vi "Mining and Dumping_r2.vi"() -> ()   [LabVIEW 2015]
uses:
  <vilib>/myRIO/Instrument Drivers/Onboard IO/PWM/typedefs/PWM Reference.ctl
  <vilib>/myRIO/Common/Instrument Driver Framework/Utilities/typedefs/myRIO Generic Hardware Reference.ctl
  <vilib>/myRIO/Common/Instrument Driver Framework/Utilities/typedefs/Hardware Version Enum.ctl
  <vilib>/myRIO/Common/Instrument Driver Framework/Utilities/typedefs/myRIO v1.0 Reference.ctl
  <vilib>/myRIO/Common/Instrument Driver Framework/Utilities/typedefs/Generic FPGA Reference.ctl
  <vilib>/myRIO/Common/Instrument Driver Framework/myRIO v1.0/PWM/typedefs/PWM Channels Enum.ctl
  <vilib>/myRIO/Instrument Drivers/Onboard IO/PWM/typedefs/PWM Configuration.ctl
  <vilib>/userdefined/High Color/nirio_resource_hc.ctl
  <vilib>/myRIO/Instrument Drivers/Onboard IO/AI/typedefs/AI Reference.ctl
  <vilib>/myRIO/Common/Instrument Driver Framework/myRIO v1.0/AI/typedefs/AI Channels List.ctl
  <vilib>/myRIO/Common/Instrument Driver Framework/myRIO v1.0/AI/typedefs/AI Channels Enum.ctl
  <vilib>/myRIO/Common/Instrument Driver Framework/Utilities/typedefs/Analog Scaling Constants List.ctl
  <vilib>/myRIO/Common/Instrument Driver Framework/Utilities/typedefs/Analog Scaling Constants.ctl
  <vilib>/myRIO/Common/Instrument Driver Framework/Utilities/vis/Is FPGA Ref Available.vi
  <vilib>/myRIO/Common/Instrument Driver Framework/myRIO v1.0/PWM/vis/myRIO v1.1 Open PWM.vi
  <vilib>/myRIO/Instrument Drivers/Onboard IO/PWM/vis/Set Duty Cycle and Frequency.vi
  <vilib>/myRIO/Common/Instrument Driver Framework/myRIO v1.0/AI/vis/myRIO v1.1 Open AI.vi
  <vilib>/myRIO/Instrument Drivers/Onboard IO/AI/vis/Read.vi
  <vilib>/myRIO/Common/Instrument Driver Framework/Utilities/vis/Validate Channels.vi
  <vilib>/myRIO/Common/Instrument Driver Framework/myRIO v1.0/PWM/vis/myRIO v1.0 Reserve PWM.vi
  <vilib>/myRIO/Common/Instrument Driver Framework/myRIO v1.0/AI/vis/myRIO v1.0 Reserve AI.vi
  <vilib>/myRIO/Common/Instrument Driver Framework/myRIO v1.0/PWM/vis/myRIO v1.0 Build MUX Configuration PWM.vi
  <vilib>/myRIO/Common/Instrument Driver Framework/myRIO v1.0/Resource Manager/vis/myRIO v1.0 Reserve Channel List.vi
  <vilib>/myRIO/Common/Instrument Driver Framework/myRIO v1.0/AI/vis/myRIO v1.0 Build MUX Configuration AI.vi
  <vilib>/myRIO/Common/Instrument Driver Framework/myRIO v1.0/Resource Manager/vis/myRIO v1.0 Create Configuration List.vi
  <vilib>/myRIO/Common/Instrument Driver Framework/myRIO v1.0/Resource Manager/vis/myRIO v1.0 Reserve Channel.vi
  <vilib>/myRIO/Common/Instrument Driver Framework/myRIO v1.0/Resource Manager/vis/myRIO v1.0 Unreserve Channel.vi
  <vilib>/myRIO/Common/Instrument Driver Framework/myRIO v1.0/Resource Manager/vis/myRIO v1.0 Build Mutex Name.vi
  <vilib>/Utility/VariantDataType/GetNumericInfo.vi
  <vilib>/Utility/error.llb/Error Cluster From Error Code.vi
  <vilib>/myRIO/Common/Instrument Driver Framework/myRIO v1.0/myRIO v1.1 Open.vi
  <vilib>/myRIO/Common/Instrument Driver Framework/Utilities/vis/IO Manager.vi
  <vilib>/myRIO/Common/Instrument Driver Framework/Utilities/vis/Configuration Manager.vi
  <vilib>/myRIO/Common/Instrument Driver Framework/myRIO v1.0/Resource Manager/vis/myRIO v1.0 Configure IO.vi
  <vilib>/myRIO/Common/Instrument Driver Framework/myRIO v1.0/myRIO v1.0 Close.vi
  <vilib>/myRIO/Common/Instrument Driver Framework/myRIO v1.0/PWM/vis/myRIO v1.0 Write PWM.vi
  <vilib>/myRIO/Common/Instrument Driver Framework/myRIO v1.0/AI/vis/myRIO v1.0 Get Scaling Constants AI.vi
  <vilib>/myRIO/Common/Instrument Driver Framework/myRIO v1.0/AI/vis/myRIO v1.0 Read AI.vi
  <vilib>/myRIO/Express VI/Onboard IO/PWM/PWM Express VI.xnode
  <vilib>/myRIO/Instrument Drivers/Onboard IO/PWM/vis/myRIO PWM Open.xnode
  <vilib>/myRIO/Express VI/Onboard IO/AI/AI Express VI.xnode
  <vilib>/myRIO/Instrument Drivers/Onboard IO/AI/vis/myRIO AI Open.xnode
  <vilib>/myRIO/Instrument Drivers/Onboard IO/PWM/PWM.lvlib
  <vilib>/myRIO/Instrument Drivers/Onboard IO/AI/AI.lvlib
panel:
  in  "Stop":bool
  out "Servo Positioin 2":dbl
  out "Servo Position 1":dbl
  out "Servo Stop":i64
  out "Stop Mining":bool
  in  "Numeric":i32
  out "Full":bool
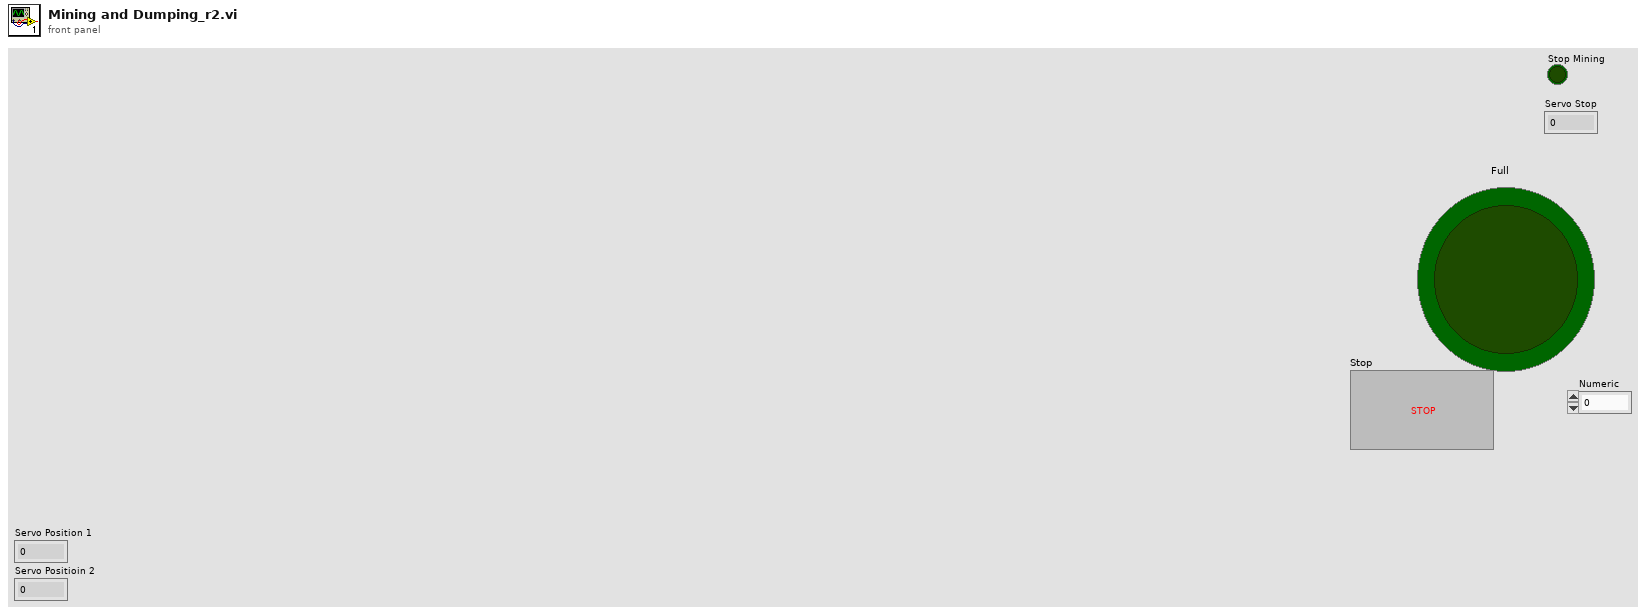
[diagram p1: front panel]
types:
  T1 = typedef "PWM.lvlib/PWM Reference.ctl" = cluster{"myRIO Reference":T2, "PWM Channels Enum":T6, "PWM Configuration":T7}
  T2 = typedef "myRIO Generic Hardware Reference.ctl" = cluster{"myRIO Model":T3, "myRIO Hardware Reference":T4}
  T3 = typedef "Hardware Version Enum.ctl" = enum16{"Unknown", "myRIO-1900", "myRIO-1950", "roboRIO"}
  T4 = typedef "myRIO v1.0 Reference.ctl" = cluster{"Generic FPGA Reference":T5, "Allow multiple opens":bool}
  T5 = typedef "Generic FPGA Reference.ctl" = refnum<k20>
  T6 = typedef "PWM Channels Enum.ctl" = enum16{"Not Connected", "C/PWM0", "C/PWM1", "A/PWM0", "A/PWM1", "A/PWM2", "B/PWM0", "B/PWM1", "B/PWM2", "PWM/PWM0", "PWM/PWM1", "PWM/PWM2", "PWM/PWM3", "PWM/PWM4", "PWM/PWM5", "PWM/PWM6", "PWM/PWM7", "PWM/PWM8", "PWM/PWM9"}
  T7 = typedef "PWM.lvlib/PWM Configuration.ctl" = cluster{"Frequency":dbl, "Duty Cycle":dbl}
  T8 = typedef "nirio_resource_hc.ctl" = tag
  T9 = typedef "AI.lvlib/AI Reference.ctl" = cluster{"myRIO Reference":T2, "AI Channels List":T10, "AI Scaling Constants List":T12}
  T10 = typedef "AI Channels List.ctl" = T11[]
  T11 = typedef "AI Channels Enum.ctl" = enum16{"Not Connected", "AudioIn/Left", "AudioIn/Right", "C/AI0", "C/AI1", "A/AI0", "A/AI1", "A/AI2", "A/AI3", "B/AI0", "B/AI1", "B/AI2", "B/AI3", "AI/AI0", "AI/AI1", "AI/AI2", "AI/AI3"}
  T12 = typedef "Analog Scaling Constants List.ctl" = T13[]
  T13 = typedef "Analog Scaling Constants.ctl" = cluster{"LSB Weight (Volts)":dbl, "Offset (Volts)":dbl, "Signed?":bool}
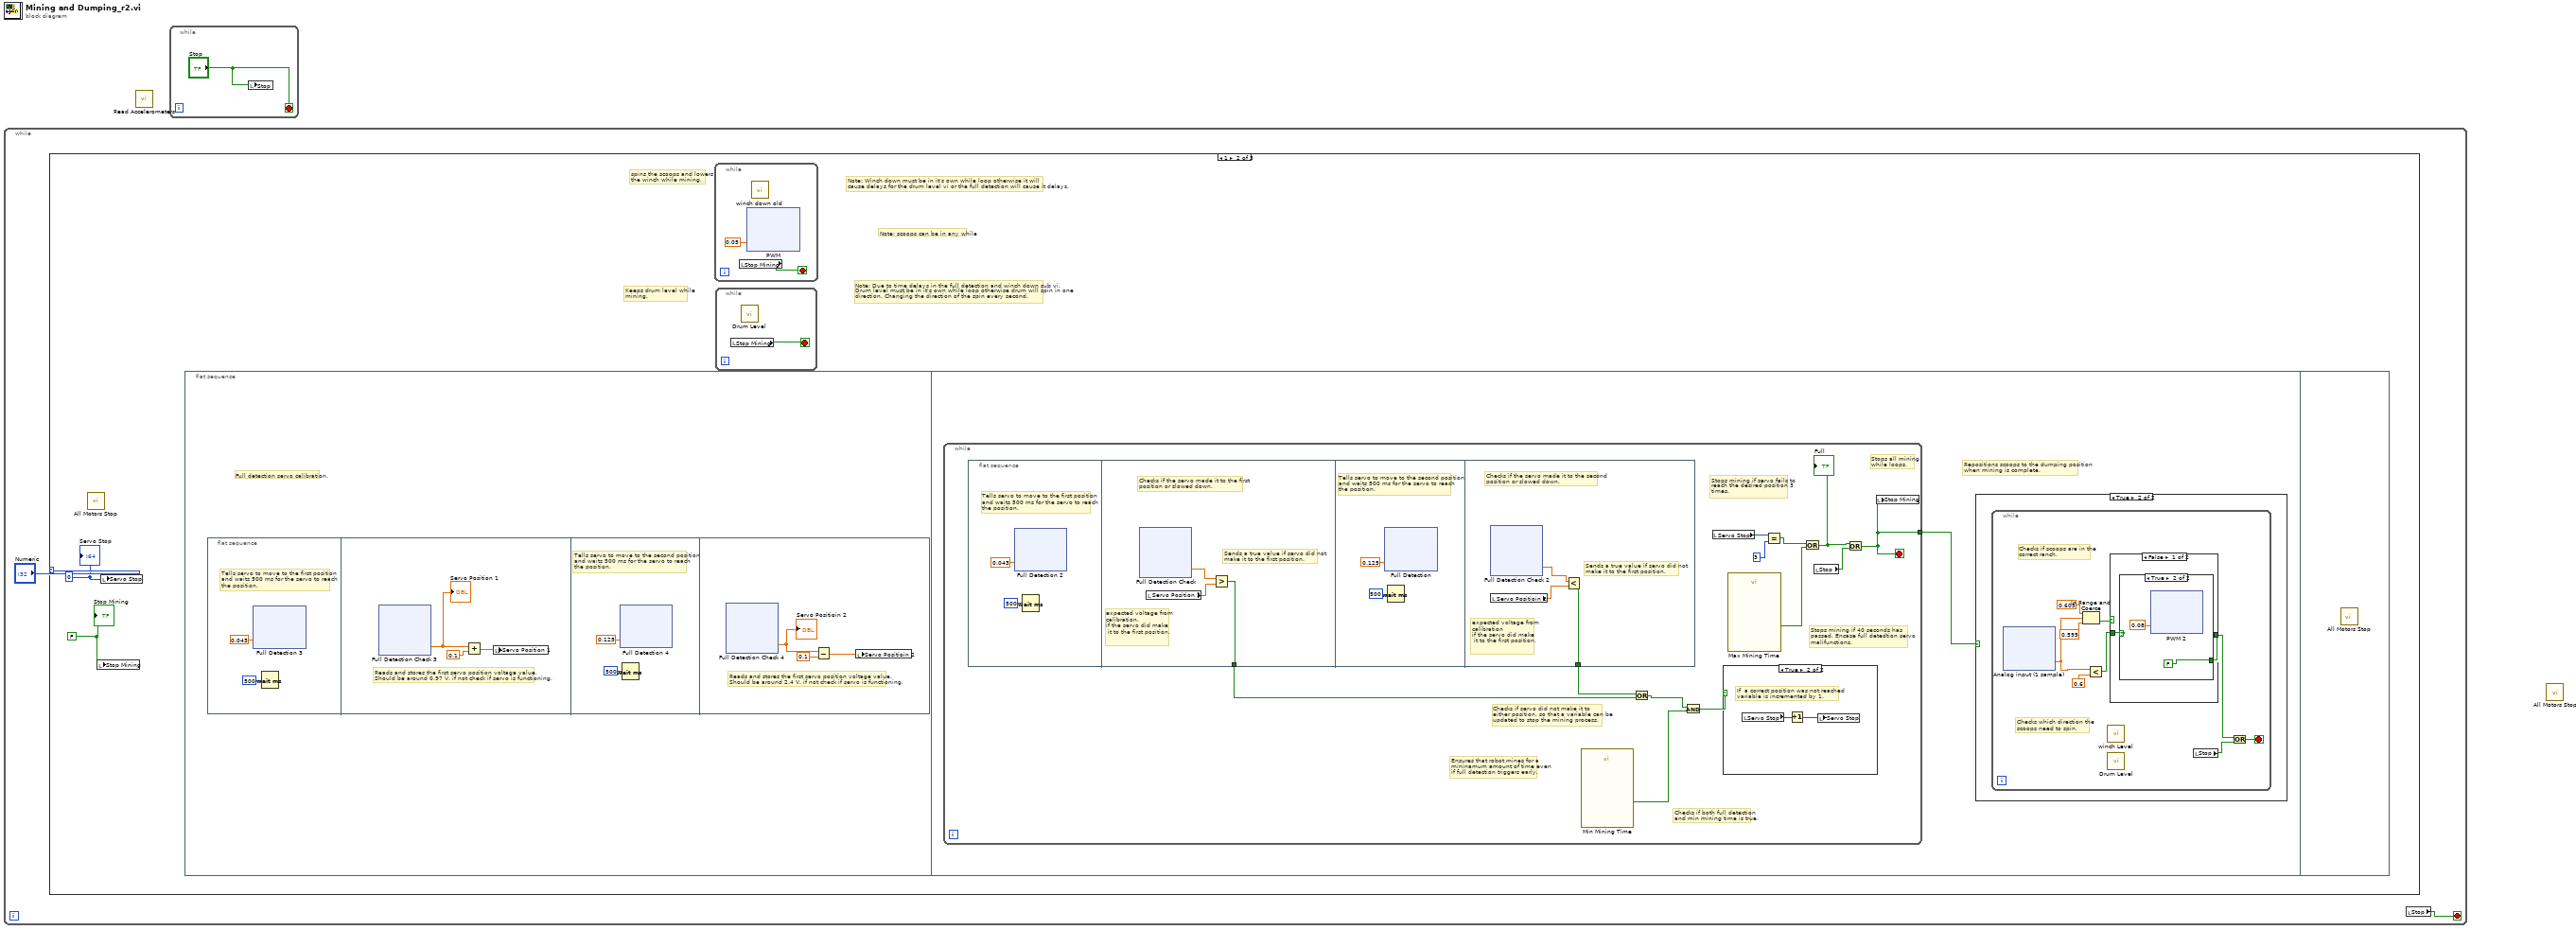
[diagram p0: block diagram]
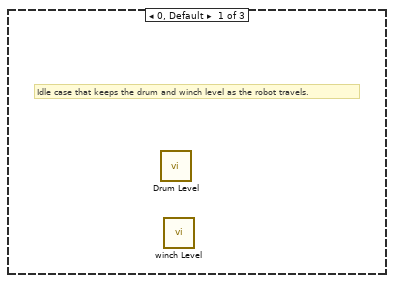
[diagram p2: hidden frame]
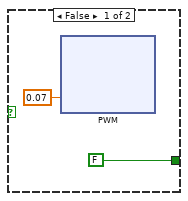
[diagram p4: hidden frame]
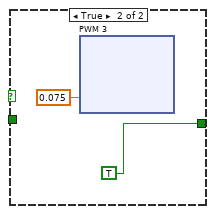
[diagram p5: hidden frame]
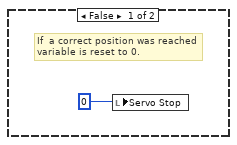
[diagram p6: hidden frame]
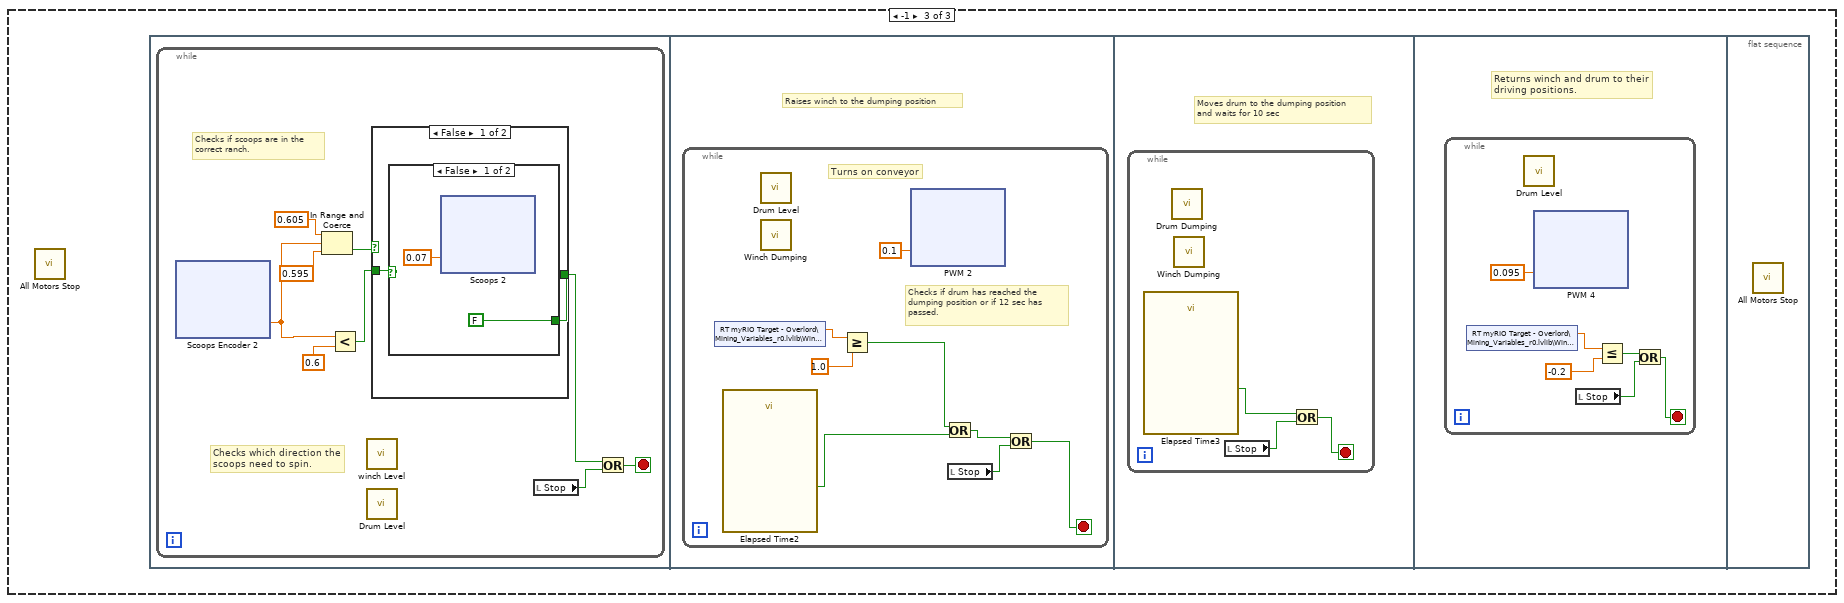
[diagram p7: hidden frame]
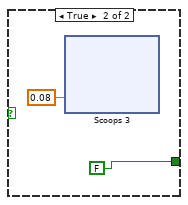
[diagram p8: hidden frame]
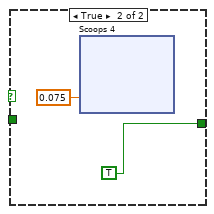
[diagram p9: hidden frame]
diagram:
  n1 = while {
    stop <- w1 stop-if-true
    n2 = case shown="1" "Numeric" {
      frame 0, Default {
        # "Idle case that keeps the drum and winch level as the robot travels."
        n3 = call "Drum Level.vi"() -> ()  [unwired: 12 in]
        n4 = call "winch Level.vi"() -> ()  [unwired: 12 in]
      }
      frame 1 {
        w4 = FALSE ("Stop")
        w3 = i64 0 ("Servo Stop")
        # "Note: scoops can be in any while"
        # "Note: Winch down must be in it's own while loop otherwise it will \ncause delays for the drum level vi or the full detection will cause it delays."
        # "Note: Due to time delays in the full detection and winch down sub vi.\nDrum level must be in it's own while loop otherwise drum will spin in one\ndirection. Changing the direction of the spin every second."
        # "spins the scoops and lowers\nthe winch while mining."
        # "Keeps drum level while \nmining."
        n5 = call "All Motors Stop.vi"() -> ()  [unwired: 12 in]
        n6 = local write "Stop Mining"(w4) -> ()
        n7 = local write "Servo Stop"(w3) -> ()
        n8 = flat-sequence {
          frame #0 {
            # "Full detection servo calibration."
            n9 = flat-sequence {
              frame #0 {
                # "Tells servo to move to the first position\nand waits 500 ms for the servo to reach \nthe position."
                n10 = xnode "Full Detection 3"("Duty Cycle"=0.043) -> ()  [unwired: 1 in, 1 out]
                n11 = Wait (ms)(milliseconds to wait=u32 500) -> ()  [unwired: 1 out]
              }
              frame #1 {
                # "Reads and stores the first servo position voltage value. \nShould be around 0.97 V. if not check if servo is functioning."
                n12 = xnode "Full Detection Check 3"() -> ("A/AI0 (Pin 3)"=w80:dbl)  [unwired: 1 in, 1 out]
                "Servo Position 1" <- w80
                n13 = Add(x=w80, y=0.1) -> (x+y=w81:dbl)
                n14 = local write "Servo Position 1"(w81) -> ()
              }
              frame #2 {
                # "Tells servo to move to the second position\nand waits 500 ms for the servo to reach \nthe position."
                n15 = xnode "Full Detection 4"("Duty Cycle"=0.125) -> ()  [unwired: 1 in, 1 out]
                n16 = Wait (ms)(milliseconds to wait=u32 500) -> ()  [unwired: 1 out]
              }
              frame #3 {
                # "Reads and stores the first servo position voltage value. \nShould be around 2.4 V. if not check if servo is functioning."
                n17 = xnode "Full Detection Check 4"() -> ("A/AI0 (Pin 3)"=w157:dbl)  [unwired: 1 in, 1 out]
                "Servo Positioin 2" <- w157
                n18 = Subtract(x=w157, y=0.1) -> (x-y=w158:dbl)
                n19 = local write "Servo Positioin 2"(w158) -> ()
              }
            }
          }
          frame #1 {
            # "Repositions scoops to the dumping position\nwhen mining is complete."
            n20 = while {
              tunnel: [w357] -> w196
              stop <- w357 stop-if-true
              # "Stops all mining \nwhile loops."
              # "Stops mining if 40 seconds has \npassed. Encase full detedtion servo \nmalifunctions."
              # "Stops mining if servo fails to \nreach the desired position 3\ntimes."
              # "Checks if both full detection \nand min mining time is true."
              # "Ensures that robot mines for a \nmininamum amount of time even\nif full detection triggers early."
              # "Checks if servo did not make it to\neither position. so that a variable can be \nupdated to stop the mining process."
              n21 = flat-sequence {
                tunnel: [w410] -> w366
                tunnel: [w486] -> w367
                frame #0 {
                  # "Tells servo to move to the first position\nand waits 500 ms for the servo to reach \nthe position."
                  n22 = xnode "Full Detection 2"("Duty Cycle"=0.043) -> ()  [unwired: 1 in, 1 out]
                  n23 = Wait (ms)(milliseconds to wait=u32 500) -> ()  [unwired: 1 out]
                }
                frame #1 {
                  # "Sends a true value if servo did not \nmake it to the first position."
                  # "expected voltage from \ncalibration.\nif the servo did make\n it to the first position."
                  # "Checks if the servo made it to the first \nposition or slowed down."
                  n24 = xnode "Full Detection Check"() -> ("A/AI0 (Pin 3)"=w409:dbl)  [unwired: 1 in, 1 out]
                  n25 = local read "Servo Position 1"() -> (w408:dbl)
                  n26 = Greater?(x=w409, y=w408) -> (0:w410:bool)
                }
                frame #2 {
                  # "Tells servo to move to the second position\nand waits 500 ms for the servo to reach \nthe position."
                  n27 = xnode "Full Detection"("Duty Cycle"=0.125) -> ()  [unwired: 1 in, 1 out]
                  n28 = Wait (ms)(milliseconds to wait=u32 500) -> ()  [unwired: 1 out]
                }
                frame #3 {
                  # "Sends a true value if servo did not \nmake it to the first position."
                  # "expected voltage from \ncalibration\nif the servo did make\n it to the first position."
                  # "Checks if the servo made it to the second \nposition or slowed down."
                  n29 = xnode "Full Detection Check 2"() -> ("A/AI0 (Pin 3)"=w487:dbl)  [unwired: 1 in, 1 out]
                  n30 = local read "Servo Positioin 2"() -> (w485:dbl)
                  n31 = Less?(x=w487, y=w485) -> (x < y?=w486:bool)
                }
              }
              n32 = call "Min Mining Time"() -> ("Time has Elapsed"=w359:bool)  [unwired: 12 in, 7 out]
              n33 = Or(x=w367, y=w366) -> (x .or. y?=w360:bool)
              n34 = And(x=w360, y=w359) -> (x .and. y?=w361:bool)
              n35 = local read "Servo Stop"() -> (w364:i64)
              n36 = case shown="True" w361 {
                frame False {
                  # "If  a correct position was reached \nvariable is reset to 0."
                  n37 = local write "Servo Stop"(i64 0 ("Servo Stop")) -> ()
                }
                frame True {
                  # "If  a correct position was not reached \nvariable is incremented by 1."
                  n38 = local read "Servo Stop"() -> (w370:i64)
                  n39 = Increment(x=w370) -> (x+1=w369:i64)
                  n40 = local write "Servo Stop"(w369) -> ()
                }
              }
              n41 = call "Max Mining Time"() -> ("Time has Elapsed"=w363:bool)  [unwired: 12 in, 7 out]
              n42 = Equal?(x=w364, y=i64 3) -> (x = y?=w362:bool)
              n43 = Or(x=w362, y=w363) -> (x .or. y?=w358:bool)
              "Full" <- w358
              n44 = local read "Stop"() -> (w356:bool)
              n45 = Or(x=w358, y=w356) -> (x .or. y?=w357:bool)
              n46 = local write "Stop Mining"(w357) -> ()
            }
            n47 = case shown="True" w196 {
              frame False {
              }
              frame True {
                n48 = while {
                  stop <- w199 stop-if-true
                  # "Checks which direction the \nscoops need to spin."
                  # "Checks if scoops are in the\ncorrect ranch."
                  n49 = xnode "Analog input (1 sample)"() -> ("A/AI1 (Pin 5)"=w202:dbl)  [unwired: 1 in, 1 out]
                  n50 = In Range and Coerce(upper limit=0.605, x=w202, lower limit=0.595) -> (In Range?=w203:bool)  [unwired: 1 out]
                  n51 = Less?(x=w202, y=0.6) -> (x < y?=w204:bool)
                  n52 = call "winch Level.vi"() -> ()  [unwired: 12 in]
                  n53 = call "Drum Level.vi"() -> ()  [unwired: 12 in]
                  n54 = case shown="False" w203 {
                    tunnel: w204 -> [w207 _]
                    tunnel: [w206 TRUE] -> w198
                    frame False {
                      n55 = case shown="True" w207 {
                        tunnel: [FALSE FALSE] -> w206
                        frame False {
                          n56 = xnode "PWM"("Duty Cycle"=0.07) -> ()  [unwired: 1 in, 1 out]
                        }
                        frame True {
                          n57 = xnode "PWM 2"("Duty Cycle"=0.08) -> ()  [unwired: 1 in, 1 out]
                        }
                      }
                    }
                    frame True {
                      n58 = xnode "PWM 3"("Duty Cycle"=0.075) -> ()  [unwired: 1 in, 1 out]
                    }
                  }
                  n59 = local read "Stop"() -> (w197:bool)
                  n60 = Or(x=w198, y=w197) -> (x .or. y?=w199:bool)
                }
              }
            }
          }
          frame #2 {
            n61 = call "All Motors Stop.vi"() -> ()  [unwired: 12 in]
          }
        }
        n62 = while {
          stop <- w5 stop-if-true
          n63 = local read "Stop Mining"() -> (w5:bool)
          n64 = xnode "PWM"("Duty Cycle"=0.05) -> ()  [unwired: 1 in, 1 out]
          n65 = call "winch down old.vi"() -> ()  [unwired: 12 in]
        }
        n66 = while {
          stop <- w525 stop-if-true
          n67 = local read "Stop Mining"() -> (w525:bool)
          n68 = call "Drum Level.vi"() -> ()  [unwired: 12 in]
        }
        "Stop Mining" <- w4
        "Servo Stop" <- w3
      }
      frame -1 {
        n69 = call "All Motors Stop.vi"() -> ()  [unwired: 12 in]
        n70 = flat-sequence {
          frame #0 {
            n71 = while {
              stop <- w528 stop-if-true
              # "Checks which direction the \nscoops need to spin."
              # "Checks if scoops are in the\ncorrect ranch."
              n72 = xnode "Scoops Encoder 2"() -> ("A/AI1 (Pin 5)"=w531:dbl)  [unwired: 1 in, 1 out]
              n73 = In Range and Coerce(upper limit=0.605, x=w531, lower limit=0.595) -> (In Range?=w532:bool)  [unwired: 1 out]
              n74 = Less?(x=w531, y=0.6) -> (x < y?=w533:bool)
              n75 = call "winch Level.vi"() -> ()  [unwired: 12 in]
              n76 = call "Drum Level.vi"() -> ()  [unwired: 12 in]
              n77 = case shown="False" w532 {
                tunnel: w533 -> [w536 _]
                tunnel: [w535 TRUE] -> w527
                frame False {
                  n78 = case shown="False" w536 {
                    tunnel: [FALSE FALSE] -> w535
                    frame False {
                      n79 = xnode "Scoops 2"("Duty Cycle"=0.07) -> ()  [unwired: 1 in, 1 out]
                    }
                    frame True {
                      n80 = xnode "Scoops 3"("Duty Cycle"=0.08) -> ()  [unwired: 1 in, 1 out]
                    }
                  }
                }
                frame True {
                  n81 = xnode "Scoops 4"("Duty Cycle"=0.075) -> ()  [unwired: 1 in, 1 out]
                }
              }
              n82 = local read "Stop"() -> (w526:bool)
              n83 = Or(x=w527, y=w526) -> (x .or. y?=w528:bool)
            }
          }
          frame #1 {
            # "Raises winch to the dumping position"
            n84 = while {
              stop <- w686 stop-if-true
              # "Turns on conveyor"
              # "Checks if drum has reached the \ndumping position or if 12 sec has \npassed."
              n85 = shared-variable "RT myRIO Target - Overlord\\Mining_Variables_r0.lvlib\\Winch Accel x"() -> (w691:dbl)  [unwired: 1 in, 1 out]
              n86 = call "Elapsed Time2"() -> ("Time has Elapsed"=w688:bool)  [unwired: 12 in, 7 out]
              n87 = call "Drum Level.vi"() -> ()  [unwired: 12 in]
              n88 = call "Winch Dumping.vi"() -> ()  [unwired: 12 in]
              n89 = Greater Or Equal?(x=w691, y=1.0) -> (x >= y?=w689:bool)
              n90 = xnode "PWM 2"("Duty Cycle"=0.1) -> ()  [unwired: 1 in, 1 out]
              n91 = Or(x=w689, y=w688) -> (x .or. y?=w687:bool)
              n92 = local read "Stop"() -> (w685:bool)
              n93 = Or(x=w687, y=w685) -> (x .or. y?=w686:bool)
            }
          }
          frame #2 {
            # "Moves drum to the dumping position\nand waits for 10 sec"
            n94 = while {
              stop <- w730 stop-if-true
              n95 = call "Elapsed Time3"() -> ("Time has Elapsed"=w729:bool)  [unwired: 12 in, 7 out]
              n96 = call "Drum Dumping.vi"() -> ()  [unwired: 12 in]
              n97 = call "Winch Dumping.vi"() -> ()  [unwired: 12 in]
              n98 = local read "Stop"() -> (w728:bool)
              n99 = Or(x=w729, y=w728) -> (x .or. y?=w730:bool)
            }
          }
          frame #3 {
            # "Returns winch and drum to their \ndriving positions."
            n100 = while {
              stop <- w732 stop-if-true
              n101 = shared-variable "RT myRIO Target - Overlord\\Mining_Variables_r0.lvlib\\Winch Accel x"() -> (w736:dbl)  [unwired: 1 in, 1 out]
              n102 = call "Drum Level.vi"() -> ()  [unwired: 12 in]
              n103 = xnode "PWM 4"("Duty Cycle"=0.095) -> ()  [unwired: 1 in, 1 out]
              n104 = local read "Stop"() -> (w731:bool)
              n105 = Less Or Equal?(x=w736, y=-0.2) -> (x <= y?=w733:bool)
              n106 = Or(x=w733, y=w731) -> (x .or. y?=w732:bool)
            }
          }
          frame #4 {
            n107 = call "All Motors Stop.vi"() -> ()  [unwired: 12 in]
          }
        }
      }
    }
    n108 = local read "Stop"() -> (w1:bool)
  }
  n109 = call "Read Accelerometers.vi"() -> ()  [unwired: 11 in, 9 out]
  n110 = while {
    stop <- "Stop" stop-if-true
    n111 = local write "Stop"("Stop") -> ()
  }
  n112 = call "All Motors Stop.vi"() -> ()  [unwired: 12 in]
